vi "显示界面.vi"(1 "VI引用句柄":refnum<vi>, 2 "error in (no error)":cluster{"状态":bool, "代码":i32, "源":string} caption="错误输入（无错误）", 3 "状态通知器":refnum<notifier>) -> (0 "error out":cluster{"状态":bool, "代码":i32, "源":string} caption="错误输出")   [LabVIEW 2014]
uses:
  <vilib>/picture/3D Picture Control/Object/Add Object (reference).vi
  <vilib>/picture/3D Picture Control/NI_3D Picture Control.lvlib
panel:
  in  "前摄像":bool
  in  "前截图":bool
  in  "前摄像头":refnum<k7>(container)
  in  "后截图":bool
  in  "主截图":bool
  out "StartChannelRecord":bool
  in  "后录像":bool
  in  "主录像":bool
  out "布尔 2":bool
  out "布尔":bool
  in  "焦距":u8
  in  "焦点":u8
  in  "Color 2":T1={"Red"=1.0, "Green"=0.0, "Blue"=0.0, "Alpha"=1.0} caption="颜色"
  in  "缩放":dbl(knob)=2.2771854734286614 scale=0.0..10.0
  out "三维图片":refnum<vi>(3d-picture)
  out "back_camera_ip":string
  in  "后摄像头":refnum<k7>(container)
  in  "主摄像头":refnum<k7>(container)
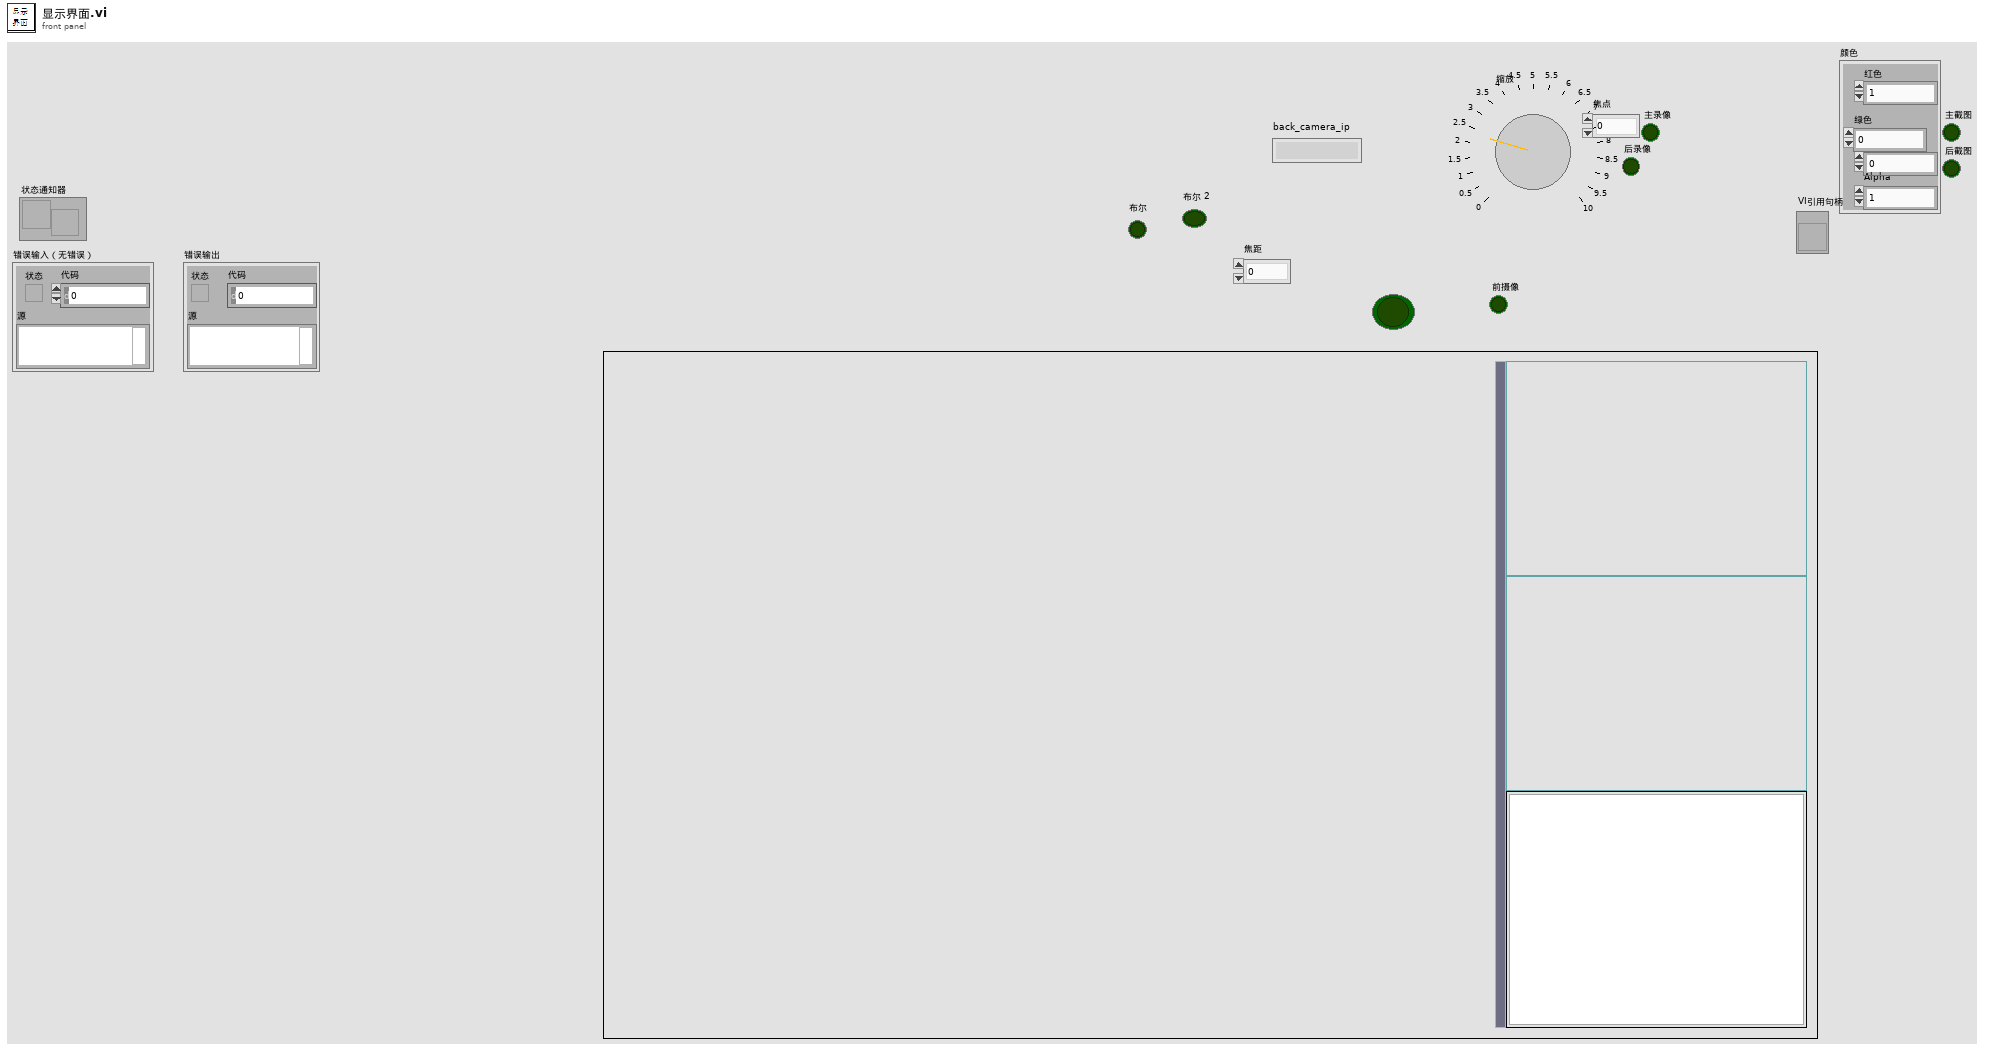
[diagram p1: front panel]
types:
  T1 = cluster{"Red":sgl, "Green":sgl, "Blue":sgl, "Alpha":sgl}
  T2 = cluster{"car_ip":u32, "car_port":i32, "wire_ip":u32, "wire_port":u32, "local_port":u32, "main_camera_ip":string, "back_camera_ip":string, "front_camera_ip":string, "car_control_ip":u32, "car_control_port":u32, "pitch":i32, "bank":i32, "heading":i32}
  T3 = enum32{"Bad", "Idle", "Run top level", "Running"}
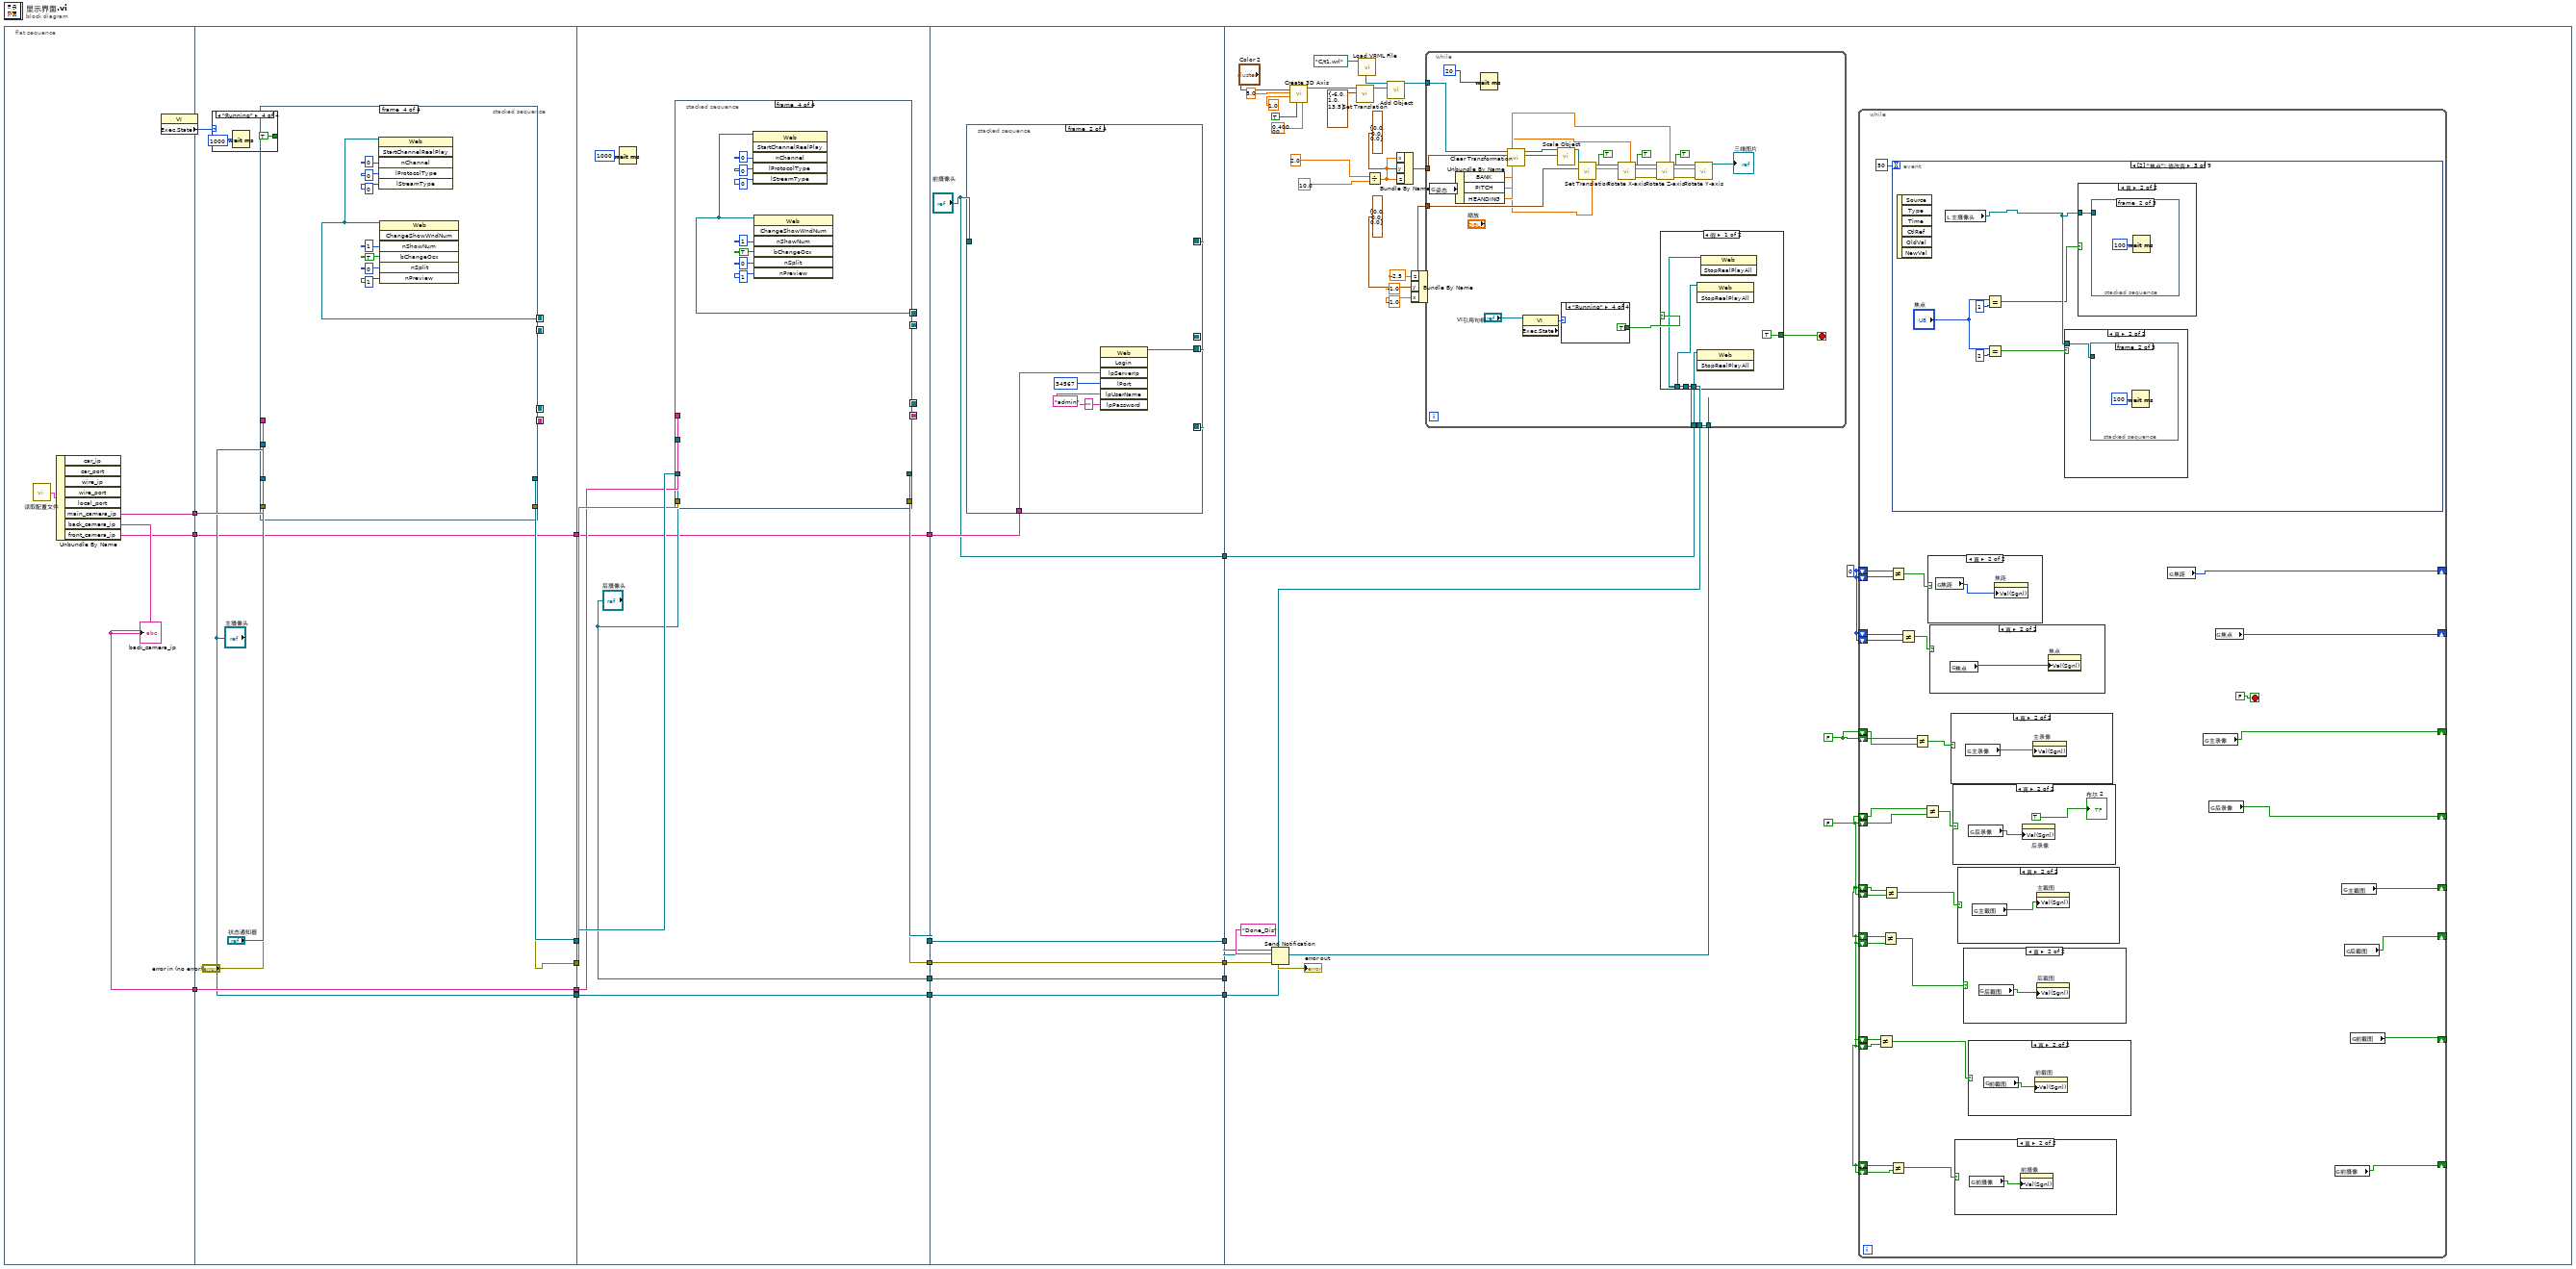
[diagram p0: block diagram]
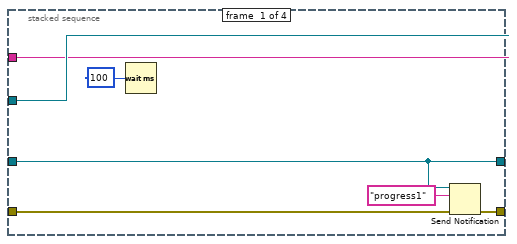
[diagram p2: hidden frame]
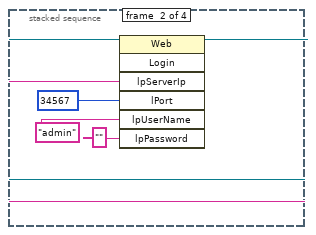
[diagram p3: hidden frame]
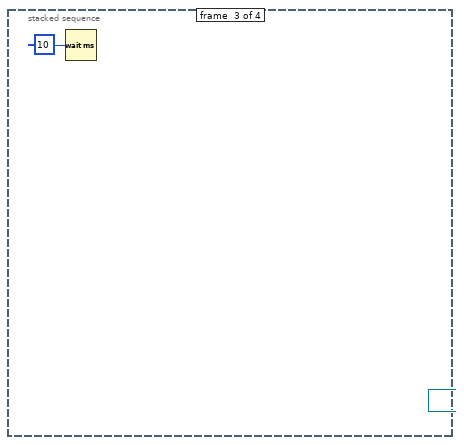
[diagram p4: hidden frame]
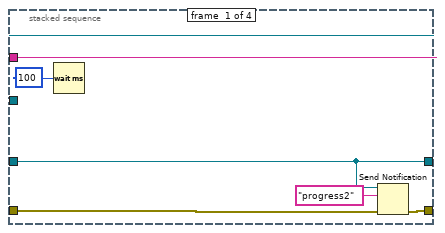
[diagram p5: hidden frame]
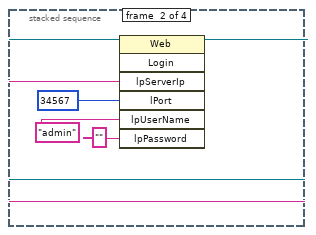
[diagram p6: hidden frame]
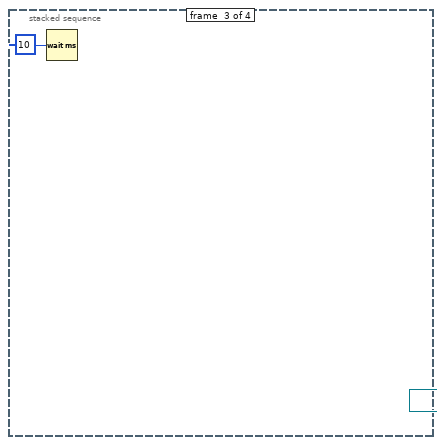
[diagram p7: hidden frame]
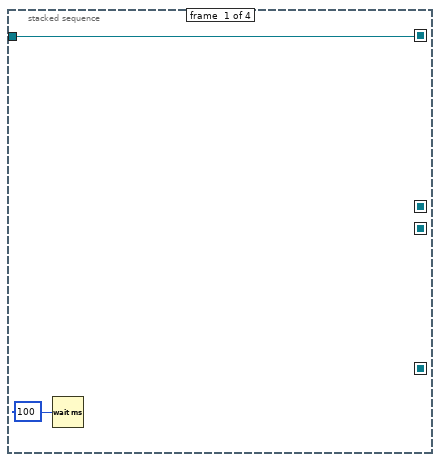
[diagram p8: hidden frame]
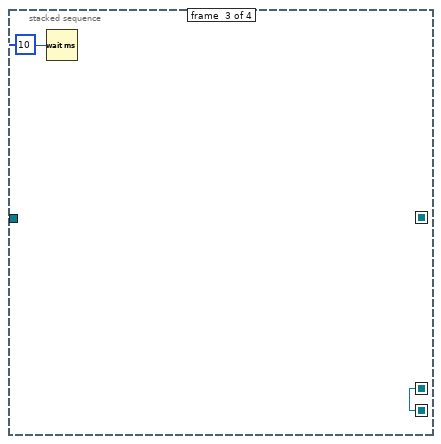
[diagram p9: hidden frame]
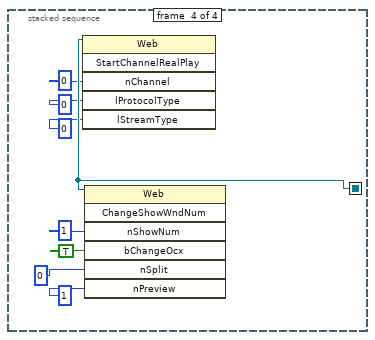
[diagram p10: hidden frame]
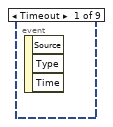
[diagram p19: hidden frame]
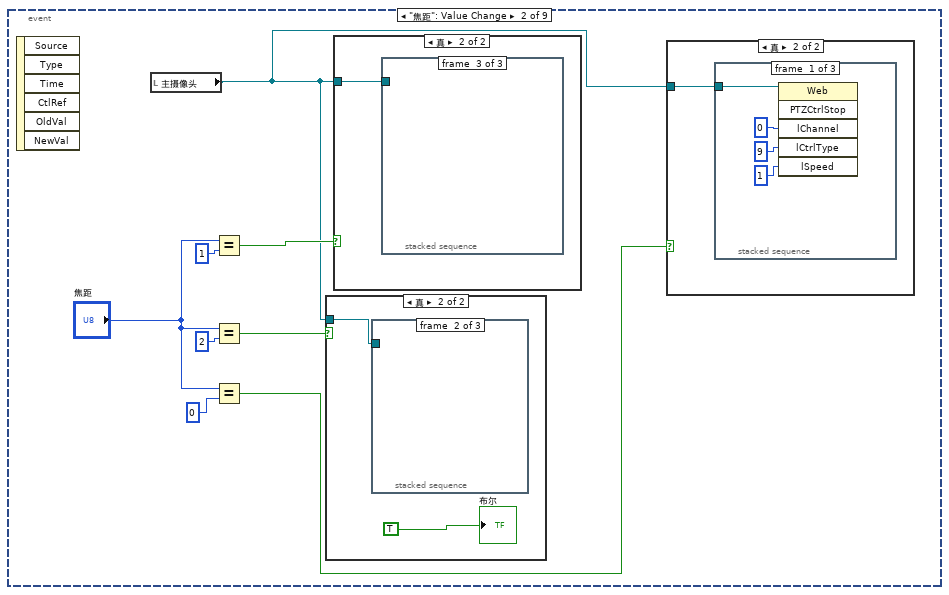
[diagram p20: hidden frame]
diagram:
  n1 = flat-sequence {
    tunnel: [w22] -> w19
    tunnel: [w21] -> w14
    tunnel: [w20] -> w2
    tunnel: w19 -> [w30]
    tunnel: [w29] -> w17
    tunnel: [w28] -> w16
    tunnel: [w27] -> w15
    tunnel: w14 -> [w27]
    tunnel: ["主摄像头"] -> w13
    tunnel: [w25] -> w3
    tunnel: w2 -> [w25]
    tunnel: w17 -> [w64]
    tunnel: [w63] -> w12
    tunnel: w16 -> [w62]
    tunnel: [w61] -> w10
    tunnel: w15 -> [w60]
    tunnel: [w59] -> w8
    tunnel: w13 -> [w59]
    tunnel: ["后摄像头"] -> w6
    tunnel: [w57] -> w4
    tunnel: w3 -> [w57]
    tunnel: w12 -> [w93]
    tunnel: [w93] -> w11
    tunnel: w10 -> [w92]
    tunnel: [w92] -> w9
    tunnel: w8 -> [w91]
    tunnel: [w91] -> w7
    tunnel: w6 -> [w90]
    tunnel: [w90] -> w5
    tunnel: w4 -> [w89]
    tunnel: ["前摄像头"] -> w1
    tunnel: w11 -> [w142]
    tunnel: w9 -> [w120]
    tunnel: w7 -> [w118]
    tunnel: w5 -> [w117]
    tunnel: w1 -> [w113]
    frame #0 {
      n2 = call "读取配置文件.vi"() -> ("簇"=w23:T2)  [unwired: 1 in]
      n3 = Unbundle By Name(w23) -> ("main_camera_ip"=w22:string, "back_camera_ip"=w21:string, "front_camera_ip"=w20:string)  [unwired: 5 out]
      "back_camera_ip" <- w21
    }
    frame #1 {
      n4 = Wait (ms)(milliseconds to wait=u32 1000 ("等待时间（毫秒）")) -> ()  [unwired: 1 out]
      n5 = stacked-sequence {
        seq-local: [w39 _ _ _] -> [_ w44 _ _]
        seq-local: [w38 _ _ _] -> [_ w43 _ _]
        seq-local: [_ w45 _ _] -> [_ _ w47 _]
        seq-local: [_ _ w47 _] -> [_ _ _ w55]
        tunnel: "主摄像头" -> [w39 _ _ _]
        tunnel: w30 -> [w38 _ _ _]
        tunnel: "状态通知器" -> [w33 _ _ _]
        tunnel: "error in (no error)" -> [w36 _ _ _]
        tunnel: [w34 _ _ _] -> w28
        tunnel: [w33 _ _ _] -> w29
        frame #0 {
          n6 = Wait (ms)(milliseconds to wait=u32 100 ("等待时间（毫秒）")) -> ()  [unwired: 1 out]
          n7 = Send Notification(notification="progress1", notifier=w33, error in (no error)=w36) -> (error out=w34:errorcluster)  [unwired: 1 out]
        }
        frame #1 {
          n8 = invoke class="Web" method="Login"(reference=w44, "lpServerIp"=w43, "lPort"=34567, "lpUserName"="admin", "lpPassword"="") -> (reference out=w45:refnum<k7>)  [unwired: 2 in, 6 out]
        }
        frame #2 {
          n9 = Wait (ms)(milliseconds to wait=u32 10 ("等待时间（毫秒）")) -> ()  [unwired: 1 out]
        }
        frame #3 {
          n10 = invoke class="Web" method="StartChannelRealPlay"(reference=w55, "nChannel"=0, "lProtocolType"=0, "lStreamType"=0) -> ()  [unwired: 2 in, 6 out]
          n11 = invoke class="Web" method="ChangeShowWndNum"(reference=w55, "nShowNum"=1, "bChangeOcx"=TRUE, "nSplit"=0, "nPreview"=1) -> ()  [unwired: 2 in, 7 out]
        }
      }
    }
    frame #2 {
      n12 = Wait (ms)(milliseconds to wait=u32 1000 ("等待时间（毫秒）")) -> ()  [unwired: 1 out]
      n13 = stacked-sequence {
        seq-local: [w71 _ _ _] -> [_ w76 _ _]
        seq-local: [w70 _ _ _] -> [_ w75 _ _]
        seq-local: [_ w77 _ _] -> [_ _ w79 _]
        seq-local: [_ _ w79 _] -> [_ _ _ w87]
        tunnel: "后摄像头" -> [w71 _ _ _]
        tunnel: w60 -> [w70 _ _ _]
        tunnel: w64 -> [w65 _ _ _]
        tunnel: w62 -> [w68 _ _ _]
        tunnel: [w66 _ _ _] -> w61
        tunnel: [w65 _ _ _] -> w63
        frame #0 {
          n14 = Wait (ms)(milliseconds to wait=u32 100 ("等待时间（毫秒）")) -> ()  [unwired: 1 out]
          n15 = Send Notification(notification="progress2", notifier=w65, error in (no error)=w68) -> (error out=w66:errorcluster)  [unwired: 1 out]
        }
        frame #1 {
          n16 = invoke class="Web" method="Login"(reference=w76, "lpServerIp"=w75, "lPort"=34567, "lpUserName"="admin", "lpPassword"="") -> (reference out=w77:refnum<k7>)  [unwired: 2 in, 6 out]
        }
        frame #2 {
          n17 = Wait (ms)(milliseconds to wait=u32 10 ("等待时间（毫秒）")) -> ()  [unwired: 1 out]
        }
        frame #3 {
          n18 = invoke class="Web" method="StartChannelRealPlay"(reference=w87, "nChannel"=0, "lProtocolType"=0, "lStreamType"=0) -> ()  [unwired: 2 in, 6 out]
          n19 = invoke class="Web" method="ChangeShowWndNum"(reference=w87, "nShowNum"=1, "bChangeOcx"=TRUE, "nSplit"=0, "nPreview"=1) -> ()  [unwired: 2 in, 7 out]
        }
      }
    }
    frame #3 {
      n20 = stacked-sequence {
        seq-local: [w94 _ _ _] -> [_ w100 _ _]
        seq-local: [_ w100 _ _] -> [_ _ w103 _]
        seq-local: [_ w100 _ _] -> [_ _ _ _]
        seq-local: [_ w101 _ _] -> [_ _ w102 _]
        seq-local: [_ _ w103 _] -> [_ _ _ w112]
        seq-local: [_ _ w102 _] -> [_ _ _ _]
        tunnel: "前摄像头" -> [w94 _ _ _]
        tunnel: w89 -> [_ w99 _ _]
        frame #0 {
          n21 = Wait (ms)(milliseconds to wait=u32 100 ("等待时间（毫秒）")) -> ()  [unwired: 1 out]
        }
        frame #1 {
          n22 = invoke class="Web" method="Login"(reference=w100, "lpServerIp"=w99, "lPort"=34567, "lpUserName"="admin", "lpPassword"="") -> (reference out=w101:refnum<k7>)  [unwired: 2 in, 6 out]
        }
        frame #2 {
          n23 = Wait (ms)(milliseconds to wait=u32 10 ("等待时间（毫秒）")) -> ()  [unwired: 1 out]
        }
        frame #3 {
          n24 = invoke class="Web" method="StartChannelRealPlay"(reference=w112, "nChannel"=0, "lProtocolType"=0, "lStreamType"=0) -> ()  [unwired: 2 in, 6 out]
          n25 = invoke class="Web" method="ChangeShowWndNum"(reference=w112, "nShowNum"=1, "bChangeOcx"=TRUE, "nSplit"=0, "nPreview"=1) -> ()  [unwired: 2 in, 7 out]
        }
      }
    }
    frame #4 {
      w114 = FALSE ("主录像")
      w115 = FALSE ("主录像")
      w116 = u8 0 ("焦点")
      n26 = Send Notification(notification="Done_Dis", notifier=w142, error in (no error)=w120) -> (error out=→"error out":errorcluster)  [unwired: 1 out]
      n27 = call <vilib>:"Create 3D Axis.vi"("Character Size"=sgl 0.4, "Axis label?"=TRUE, "Color"="Color 2", "Radius"=sgl 1.0, "Length"=sgl 5.0) -> ("New Object Refnum"=w133:refnum<vi>)  [unwired: 5 in, 1 out]
      n28 = call <vilib>:"Set Translation.vi"("Translation"=cluster{"X":sgl, "Y":sgl, "Z":sgl} {"X"=-6.0, "Y"=1.0, "Z"=13.5}, "Scene Object"=w133) -> ("Translated Object"=w132:refnum<vi>)  [unwired: 8 in, 1 out]
      n29 = call <vilib>:"Load VRML File.vi"("Path"=path "C:/t1.wrl" ("路径")) -> ("Scene:Read Scene File"=w135:refnum<vi>)  [unwired: 9 in, 1 out]
      n30 = Divide(x=2.0, y=10.0) -> (x/y=w125:dbl)
      n31 = call-poly <vilib>:"Add Object.vi"("New Object In"=w132, "Scene Object In"=w135) -> ("Scene Object Out"=w137:refnum<vi>)  [unwired: 7 in, 2 out]
      n32 = Bundle By Name(cluster=cluster{"x":dbl, "y":dbl, "z":dbl} {"x"=0.0, "y"=0.0, "z"=0.0}, "x"=w125, "y"=w125, "z"=w125) -> (w123:cluster{"x":dbl, "y":dbl, "z":dbl})
      n33 = Bundle By Name(cluster=cluster{"x":dbl, "y":dbl, "z":dbl} {"x"=0.0, "y"=0.0, "z"=0.0}, "z"=-2.5, "y"=-1.0, "x"=-1.0) -> (w130:cluster{"x":dbl, "y":dbl, "z":dbl})
      n34 = while {
        tunnel: w137 -> [w308]
        tunnel: w130 -> [w307]
        tunnel: w123 -> [w306]
        tunnel: w118 -> [w305]
        tunnel: w117 -> [w304]
        tunnel: w113 -> [w302]
        stop <- w303 stop-if-true
        n35 = global read "全局变量.vi" "姿态"() -> (w289:cluster{"PITCH":dbl, "BANK":dbl, "HEANDING":dbl})
        n36 = Unbundle By Name(w289) -> ("BANK"=w286:dbl, "PITCH"=w287:dbl, "HEANDING"=w288:dbl)
        n37 = Wait (ms)(milliseconds to wait=u32 20 ("等待时间（毫秒）")) -> ()  [unwired: 1 out]
        n38 = call <vilib>:"Clear Transformation.vi"("Object Refnum In"=w308) -> ("Object Refnum Out"=w291:refnum<vi>)  [unwired: 9 in, 1 out]
        n39 = property class="VI"(reference="VI引用句柄") -> ("Exec.State"=w285:T3)  [unwired: 1 in, 2 out]
        n40 = call <vilib>:"Scale Object.vi"("Scale"=w306, "Scene.Object In"=w291) -> ("Scene.Object Out"=w300:refnum<vi>)  [unwired: 8 in, 1 out]
        n41 = case shown="\"Running\"" w285 {
          tunnel: [FALSE FALSE TRUE TRUE] -> w283
          frame "Bad", Default {
          }
          frame "Idle" {
          }
          frame "Run top level" {
          }
          frame "Running" {
          }
        }
        n42 = call <vilib>:"Set Translation.vi"("Translation"=w307, "Scene Object"=w300) -> ("Translated Object"=w299:refnum<vi>)  [unwired: 8 in, 1 out]
        n43 = call <vilib>:"Rotate X-axis.vi"("Relative?"=TRUE, "angle"=w286, "Scene Object In"=w299) -> ("error out"=w298:errorcluster, "Scene Object Out"=w297:refnum<vi>)  [unwired: 7 in]
        n44 = call <vilib>:"Rotate Z-axis.vi"("Relative?"=TRUE, "error in (no error)"=w298, "angle"=w287, "Scene Object In"=w297) -> ("error out"=w294:errorcluster, "Scene Object Out"=w293:refnum<vi>)  [unwired: 6 in]
        n45 = case shown="假" w283 {
          tunnel: w305 -> [w315 _]
          tunnel: w304 -> [w316 _]
          tunnel: [TRUE FALSE] -> w303
          tunnel: w302 -> [w313 _]
          frame False {
            n46 = invoke class="Web" method="StopRealPlayAll"(reference=w316) -> ()  [unwired: 2 in, 3 out]
            n47 = invoke class="Web" method="StopRealPlayAll"(reference=w313) -> ()  [unwired: 2 in, 3 out]
            n48 = invoke class="Web" method="StopRealPlayAll"(reference=w315) -> ()  [unwired: 2 in, 3 out]
          }
          frame True {
          }
        }
        n49 = call <vilib>:"Rotate Y-axis.vi"("Relative?"=TRUE, "error in (no error)"=w294, "angle"=w288, "Scene Object In"=w293) -> ("Scene Object Out"=→"三维图片":refnum<vi>)  [unwired: 6 in, 1 out]
      }
      n50 = while {
        shift-right: [w175] -> _
        shift-left: w116 -> [w174]
        shift-left: w116 -> [w173]
        shift-right: [w171] -> _
        shift-left: w116 -> [w170]
        shift-left: w116 -> [w169]
        shift-right: [w167] -> _
        shift-left: w115 -> [w165]
        shift-left: w115 -> [w164]
        shift-right: [w166] -> _
        shift-left: w114 -> [w163]
        shift-left: w114 -> [w162]
        shift-right: [w155] -> _
        shift-left: w114 -> [w159]
        shift-right: [w154] -> _
        shift-left: w114 -> [w157]
        shift-left: w114 -> [w158]
        shift-left: w114 -> [w156]
        shift-right: [w148] -> _
        shift-left: w114 -> [w151]
        shift-left: w114 -> [w150]
        shift-right: [w144] -> _
        shift-left: w114 -> [w147]
        shift-left: w114 -> [w146]
        stop <- FALSE stop-if-true
        n51 = Not Equal?(x=w151, y=w150) -> (x != y?=w149:bool)
        n52 = Not Equal?(x=w157, y=w156) -> (x != y?=w152:bool)
        n53 = Not Equal?(x=w159, y=w158) -> (x != y?=w153:bool)
        n54 = Not Equal?(x=w174, y=w173) -> (x != y?=w172:bool)
        n55 = Not Equal?(x=w147, y=w146) -> (x != y?=w145:bool)
        n56 = event shown="[2] \"焦点\": 值改变" {
          selector: _ -> [_ _ _ _ _ _ _ _ _]
          dyn-events: _ -> [_ _ _ _ _ _ _ _ _]
          timeout: 50 -> [_ _ _ _ _ _ _ _ _]
          event Timeout {
            n57 = event-data() -> ()  [unwired: 1 in, 3 out]
          }
          event "焦距": Value Change {
            n58 = event-data() -> ()  [unwired: 1 in, 6 out]
            n59 = local read "主摄像头"() -> (w191:refnum<k7>)
            n60 = Equal?(x="焦距", y=u8 1) -> (x = y?=w193:bool)
            n61 = Equal?(x="焦距", y=u8 2) -> (x = y?=w190:bool)
            n62 = Equal?(x="焦距", y=u8 0) -> (x = y?=w187:bool)
            n63 = case shown="真" w190 {
              tunnel: w191 -> [_ w210]
              frame False {
              }
              frame True {
                n64 = stacked-sequence {
                  tunnel: w210 -> [w211 _ _]
                  frame #0 {
                    n65 = invoke class="Web" method="PTZCtrlStart"(reference=w211, "lChannle"=0, "lCtrlType"=8, "lSpeed"=1) -> ()  [unwired: 2 in, 6 out]
                  }
                  frame #1 {
                  }
                  frame #2 {
                  }
                }
                "布尔" <- TRUE ("布尔")
              }
            }
            n66 = case shown="真" w193 {
              tunnel: w191 -> [_ w204]
              frame False {
              }
              frame True {
                n67 = stacked-sequence {
                  tunnel: w204 -> [w205 _ _]
                  frame #0 {
                    n68 = invoke class="Web" method="PTZCtrlStart"(reference=w205, "lChannle"=0, "lCtrlType"=9, "lSpeed"=1) -> ()  [unwired: 2 in, 6 out]
                  }
                  frame #1 {
                  }
                  frame #2 {
                  }
                }
              }
            }
            n69 = case shown="真" w187 {
              tunnel: w191 -> [_ w195]
              frame False {
              }
              frame True {
                n70 = stacked-sequence {
                  tunnel: w195 -> [w196 _ w200]
                  frame #0 {
                    n71 = invoke class="Web" method="PTZCtrlStop"(reference=w196, "lChannel"=0 ("lChannle"), "lCtrlType"=9, "lSpeed"=1) -> ()  [unwired: 2 in, 6 out]
                  }
                  frame #1 {
                  }
                  frame #2 {
                    n72 = invoke class="Web" method="PTZCtrlStop"(reference=w200, "lChannel"=0, "lCtrlType"=8, "lSpeed"=1) -> ()  [unwired: 2 in, 6 out]
                  }
                }
              }
            }
          }
          event "焦点": Value Change {
            n73 = event-data() -> ()  [unwired: 1 in, 6 out]
            n74 = local read "主摄像头"() -> (w216:refnum<k7>)
            n75 = Equal?(x="焦点", y=u8 1) -> (x = y?=w215:bool)
            n76 = Equal?(x="焦点", y=u8 2) -> (x = y?=w218:bool)
            n77 = case shown="真" w218 {
              tunnel: w216 -> [_ w231]
              frame False {
              }
              frame True {
                n78 = stacked-sequence {
                  tunnel: w231 -> [w232 _ w237]
                  frame #0 {
                    n79 = invoke class="Web" method="PTZCtrlStart"(reference=w232, "lChannle"=0, "lCtrlType"=11, "lSpeed"=1) -> ()  [unwired: 2 in, 6 out]
                  }
                  frame #1 {
                    n80 = Wait (ms)(milliseconds to wait=u32 100 ("等待时间（毫秒）")) -> ()  [unwired: 1 out]
                  }
                  frame #2 {
                    n81 = invoke class="Web" method="PTZCtrlStop"(reference=w237, "lChannel"=0, "lCtrlType"=11, "lSpeed"=1) -> ()  [unwired: 2 in, 6 out]
                  }
                }
              }
            }
            n82 = case shown="真" w215 {
              tunnel: w216 -> [_ w221]
              frame False {
              }
              frame True {
                n83 = stacked-sequence {
                  tunnel: w221 -> [w222 _ w227]
                  frame #0 {
                    n84 = invoke class="Web" method="PTZCtrlStart"(reference=w222, "lChannle"=0, "lCtrlType"=10, "lSpeed"=1) -> ()  [unwired: 2 in, 6 out]
                  }
                  frame #1 {
                    n85 = Wait (ms)(milliseconds to wait=u32 100 ("等待时间（毫秒）")) -> ()  [unwired: 1 out]
                  }
                  frame #2 {
                    n86 = invoke class="Web" method="PTZCtrlStop"(reference=w227, "lChannel"=0, "lCtrlType"=10, "lSpeed"=1) -> ()  [unwired: 2 in, 6 out]
                  }
                }
              }
            }
          }
          event "主录像": Value Change {
            n87 = event-data() -> ()  [unwired: 1 in, 6 out]
            n88 = local read "主摄像头"() -> (w241:refnum<k7>)
            n89 = case shown="真" "主录像" {
              tunnel: w241 -> [w244 w247]
              frame False {
                n90 = invoke class="Web" method="StopChannelRecord"(reference=w244, "nChannel"=0) -> ()  [unwired: 2 in, 4 out]
              }
              frame True {
                n91 = invoke class="Web" method="StartChannelRecord"(reference=w247, "nChannel"=0, "lpSaveFile"="D:\\main_record", "nType"=0) -> ()  [unwired: 2 in, 6 out]
              }
            }
          }
          event "前摄像": Value Change {
            n92 = event-data() -> ()  [unwired: 1 in, 6 out]
            n93 = local read "前摄像头"() -> (w249:refnum<k7>)
            n94 = case shown="真" "前摄像" {
              tunnel: w249 -> [w252 w255]
              frame False {
                n95 = invoke class="Web" method="StopChannelRecord"(reference=w252, "nChannel"=0) -> ()  [unwired: 2 in, 4 out]
              }
              frame True {
                n96 = invoke class="Web" method="StartChannelRecord"(reference=w255, "nChannel"=0, "lpSaveFile"="D:\\fornt_record", "nType"=0) -> ()  [unwired: 2 in, 6 out]
              }
            }
          }
          event "后录像": Value Change {
            n97 = event-data() -> ()  [unwired: 1 in, 6 out]
            n98 = local read "后摄像头"() -> (w257:refnum<k7>)
            n99 = case shown="真" "后录像" {
              tunnel: w257 -> [w262 w266]
              tunnel: [w260 w263] -> w259
              frame False {
                n100 = invoke class="Web" method="StopChannelRecord"(reference=w262, "nChannel"=0) -> ("StopChannelRecord"=w260:bool)  [unwired: 2 in, 3 out]
              }
              frame True {
                n101 = invoke class="Web" method="StartChannelRecord"(reference=w266, "nChannel"=0, "lpSaveFile"="D:\\back_record", "nType"=0) -> ("StartChannelRecord"=w263:bool)  [unwired: 2 in, 5 out]
              }
            }
            "StartChannelRecord" <- w259
          }
          event "主截图": Value Change {
            n102 = event-data() -> ()  [unwired: 1 in, 6 out]
            n103 = local read "主摄像头"() -> (w268:refnum<k7>)
            n104 = case shown="真" "主截图" {
              tunnel: w268 -> [_ w270]
              frame False {
              }
              frame True {
                n105 = invoke class="Web" method="BMPChannelCapturePicture"(reference=w270, "nChannel"=0, "lpSaveFile"="D:\\main_record") -> ()  [unwired: 2 in, 5 out]
              }
            }
          }
          event "前截图": Value Change {
            n106 = event-data() -> ()  [unwired: 1 in, 6 out]
            n107 = local read "前摄像头"() -> (w273:refnum<k7>)
            n108 = case shown="真" "前截图" {
              tunnel: w273 -> [_ w275]
              frame False {
              }
              frame True {
                n109 = invoke class="Web" method="BMPChannelCapturePicture"(reference=w275, "nChannel"=0, "lpSaveFile"="D:\\main_record") -> ()  [unwired: 2 in, 5 out]
              }
            }
          }
          event "后截图": Value Change {
            n110 = event-data() -> ()  [unwired: 1 in, 6 out]
            n111 = local read "后摄像头"() -> (w279:refnum<k7>)
            n112 = case shown="真" "后截图" {
              tunnel: w279 -> [_ w280]
              frame False {
              }
              frame True {
                n113 = invoke class="Web" method="BMPChannelCapturePicture"(reference=w280, "nChannel"=0, "lpSaveFile"="D:\\main_record") -> ()  [unwired: 2 in, 5 out]
              }
            }
          }
        }
        n114 = Not Equal?(x=w170, y=w169) -> (x != y?=w168:bool)
        n115 = Not Equal?(x=w165, y=w164) -> (x != y?=w161:bool)
        n116 = Not Equal?(x=w163, y=w162) -> (x != y?=w160:bool)
        n117 = case shown="真" w172 {
          frame False {
          }
          frame True {
            n118 = global read "全局变量.vi" "焦距"() -> (w186:u8)
            n119 = property on="焦距" class="DigNum (严格)"("Val(Sgnl)"=w186) -> ()  [unwired: 2 in, 2 out]
          }
        }
        n120 = case shown="真" w168 {
          frame False {
          }
          frame True {
            n121 = global read "全局变量.vi" "焦点"() -> (w185:u8)
            n122 = property on="焦点" class="DigNum (严格)"("Val(Sgnl)"=w185) -> ()  [unwired: 2 in, 2 out]
          }
        }
        n123 = case shown="真" w161 {
          frame False {
          }
          frame True {
            n124 = global read "全局变量.vi" "主录像"() -> (w184:bool)
            n125 = property on="主录像" class="Bool (严格)"("Val(Sgnl)"=w184) -> ()  [unwired: 2 in, 2 out]
          }
        }
        n126 = case shown="真" w160 {
          frame False {
          }
          frame True {
            n127 = global read "全局变量.vi" "后录像"() -> (w183:bool)
            n128 = property on="后录像" class="Bool (严格)"("Val(Sgnl)"=w183) -> ()  [unwired: 2 in, 2 out]
            "布尔 2" <- TRUE ("布尔")
          }
        }
        n129 = case shown="真" w145 {
          frame False {
          }
          frame True {
            n130 = global read "全局变量.vi" "前摄像"() -> (w178:bool)
            n131 = property on="前摄像" class="Bool (严格)"("Val(Sgnl)"=w178) -> ()  [unwired: 2 in, 2 out]
          }
        }
        n132 = case shown="真" w153 {
          frame False {
          }
          frame True {
            n133 = global read "全局变量.vi" "主截图"() -> (w181:bool)
            n134 = property on="主截图" class="Bool (严格)"("Val(Sgnl)"=w181) -> ()  [unwired: 2 in, 2 out]
          }
        }
        n135 = case shown="真" w152 {
          frame False {
          }
          frame True {
            n136 = global read "全局变量.vi" "后截图"() -> (w180:bool)
            n137 = property on="后截图" class="Bool (严格)"("Val(Sgnl)"=w180) -> ()  [unwired: 2 in, 2 out]
          }
        }
        n138 = case shown="真" w149 {
          frame False {
          }
          frame True {
            n139 = global read "全局变量.vi" "前截图"() -> (w179:bool)
            n140 = property on="前截图" class="Bool (严格)"("Val(Sgnl)"=w179) -> ()  [unwired: 2 in, 2 out]
          }
        }
        n141 = global read "全局变量.vi" "焦距"() -> (w175:u8)
        n142 = global read "全局变量.vi" "主录像"() -> (w167:bool)
        n143 = global read "全局变量.vi" "后录像"() -> (w166:bool)
        n144 = global read "全局变量.vi" "焦点"() -> (w171:u8)
        n145 = global read "全局变量.vi" "前摄像"() -> (w144:bool)
        n146 = global read "全局变量.vi" "主截图"() -> (w155:bool)
        n147 = global read "全局变量.vi" "后截图"() -> (w154:bool)
        n148 = global read "全局变量.vi" "前截图"() -> (w148:bool)
      }
    }
  }
  n149 = property class="VI"() -> ("Exec.State"=w18:T3)  [unwired: 2 in, 2 out]
  n150 = case shown="\"Running\"" w18 {
    tunnel: [FALSE FALSE TRUE TRUE] -> _
    frame "Bad", Default {
    }
    frame "Idle" {
    }
    frame "Run top level" {
    }
    frame "Running" {
    }
  }
